vi "WaveformData.vi"() -> ()   [LabVIEW 2020]
panel:
  out "Graph Data":waveform(dbl)[](array[waveform])
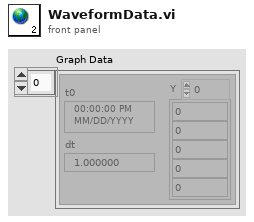
[diagram p1: front panel]
diagram:
